vi "Shutdown Master.vi"(8 "error in":errorcluster, 11 "TCP master in":refnum<class "TCP Master.lvclass">) -> (0 "error out":errorcluster, 3 "TCP master out":refnum<class "TCP Master.lvclass">)   [LabVIEW 2021, in "TCP Master.lvclass"]
doc: "Closes the TCP connection stored in the class."
uses:
  TCP Master.lvclass
  TCP Master.lvclass/TCP Master.ctl
  Network Protocol.lvclass
  Transmission Data Unit/Transmission Data Unit.lvclass
  D:/my_projects/projects/Algorithms/Labview/21/Modbus_v121c/Network Protocol/Network Master/Network Master.lvclass
  D:/my_projects/projects/Algorithms/Labview/21/Modbus_v121c/Network Protocol/Network Protocol.lvclass
  D:/my_projects/projects/Algorithms/Labview/21/Modbus_v121c/Network Protocol/Network Master/TCP/TCP Master.lvclass
  Network Interface/Network Interface.lvclass
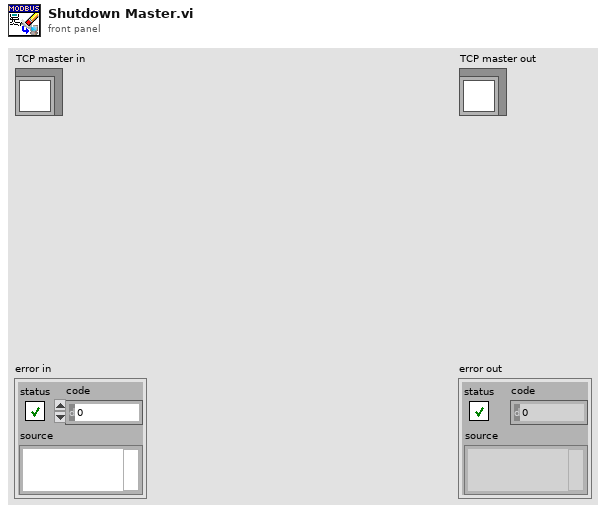
[diagram p1: front panel]
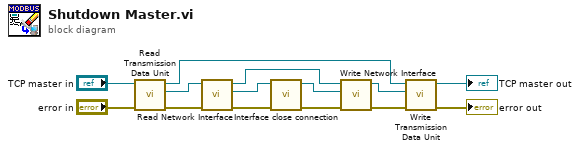
[diagram p0: block diagram]
diagram:
  n1 = call "Read Transmission Data Unit.vi"("error in (no error)"="error in", "Network Protocol in"="TCP master in") -> ("error out"=w9:errorcluster, "Transmission Data Unit"=w14:refnum<class "Transmission Data Unit.lvclass">, "Network Protocol out"=w5:refnum<class "TCP Master.lvclass">)  [unwired: 7 in]
  n2 = call "Read Network Interface.vi"("error in (no error)"=w9, "Transmission Data Unit in"=w14) -> ("error out"=w8:errorcluster, "Network Interface"=w13:refnum<class "Network Interface.lvclass">, "Transmission Data Unit out"=w10:refnum<class "Transmission Data Unit.lvclass">)  [unwired: 7 in]
  n3 = call-dynamic "Interface close connection.vi"("error in"=w8, "interface in"=w13) -> ("error out"=w7:errorcluster, "interface out"=w12:refnum<class "Network Interface.lvclass">)  [unwired: 8 in]
  n4 = call "Write Network Interface.vi"("error in (no error)"=w7, "Network Interface"=w12, "Transmission Data Unit in"=w10) -> ("error out"=w6:errorcluster, "Transmission Data Unit out"=w11:refnum<class "Transmission Data Unit.lvclass">)  [unwired: 7 in]
  n5 = call "Write Transmission Data Unit.vi"("error in (no error)"=w6, "Transmission Data Unit"=w11, "Network Protocol in"=w5) -> ("error out"=→"error out":errorcluster, "Network Protocol out"=→"TCP master out":refnum<class "TCP Master.lvclass">)  [unwired: 7 in]
